vi "FlatToRichcrio_dashboard_ShutdownRequest.vi"(5 "OutputClusterType":T1, 11 "InputCluster":T2) -> (3 "OutputCluster":T1)   [LabVIEW 2026, in "WebPageInterface_client.lvlib"]
uses:
  WebPageInterface_client.lvlib
  crio_dashboard_ShutdownRequest.ctl
  crio_dashboard_ShutdownRequest_Flat.ctl
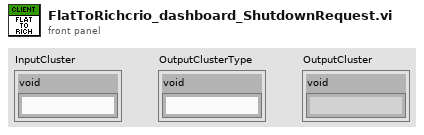
[diagram p1: front panel]
types:
  T1 = typedef "WebPageInterface_client.lvlib/crio_dashboard_ShutdownRequest.ctl" = cluster{"void":string}
  T2 = typedef "WebPageInterface_client.lvlib/crio_dashboard_ShutdownRequest_Flat.ctl" = cluster{"void":string}
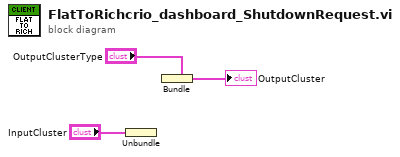
[diagram p0: block diagram]
diagram:
  n1 = Unbundle "Unbundle"("InputCluster") -> ()  [unwired: 1 out]
  n2 = Bundle "Bundle"(cluster="OutputClusterType") -> (→"OutputCluster":T1)  [unwired: 1 in]
